vi "Write BRAND SELECTED.vi"(8 "error in (no error)":errorcluster, 10 "BRAND SELECTED":enum16{"NXP", "CYPRESS", "SIMULATED"}(ring), 11 "Serial Devices in":refnum<class "Serial Devices.lvclass">) -> (0 "error out":errorcluster, 3 "Serial Devices out":refnum<class "Serial Devices.lvclass">)   [LabVIEW 2019, in "Serial Devices.lvlib" / "Serial Devices.lvclass"]
uses:
  Serial Devices.lvclass
  Serial Devices.lvclass/Serial Devices.ctl
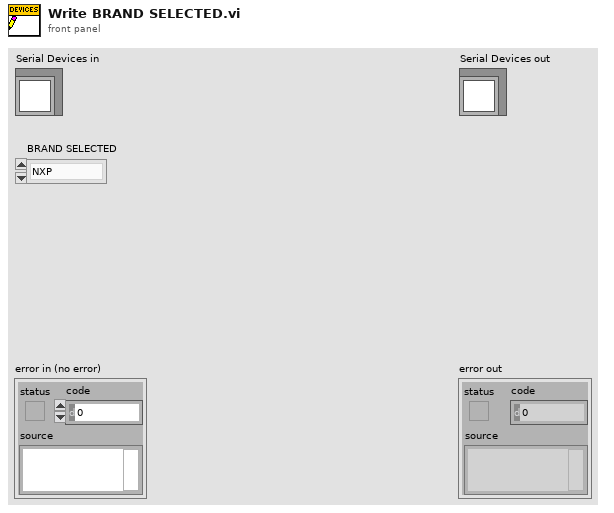
[diagram p1: front panel]
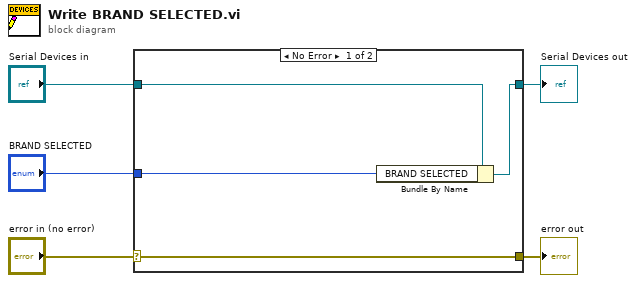
[diagram p0: block diagram]
diagram:
  n1 = case shown="No Error" "error in (no error)" {
    selector: "error in (no error)" -> [w9 w10]
    tunnel: [w9 w10] -> w4
    tunnel: [w7 w11] -> w2
    tunnel: "Serial Devices in" -> [w8 w11]
    tunnel: "BRAND SELECTED" -> [w6 _]
    frame No Error {
      n2 = Bundle By Name(cluster=w8, "BRAND SELECTED"=w6) -> (w7:refnum<class "Serial Devices.lvclass">)
    }
    frame Error {
    }
  }
  "error out" <- w4
  "Serial Devices out" <- w2
